vi "NI VeriStand - Save Configuration File.vi"(8 "Error in":errorcluster, 11 "Runtime Configuration Ref in":refnum<k39>) -> (0 "Error out":errorcluster, 2 "Success":bool, 3 "Runtime Configuration Ref out":refnum<k39>)   [LabVIEW 2027, in "Runtime Configuration File API.lvlib"]
uses:
  Runtime Configuration File API.lvlib
  C:/NetCoreDLL/NationalInstruments.VeriStand.SystemDefinitionAPI.dll
  NetCoreDLL/NationalInstruments.VeriStand.SystemDefinitionAPI.dll
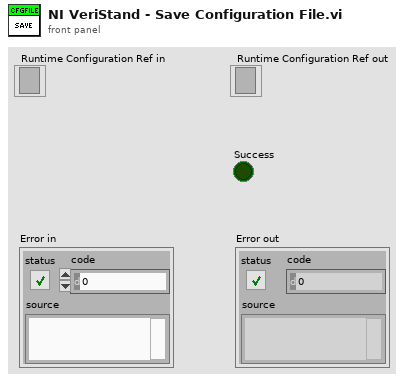
[diagram p1: front panel]
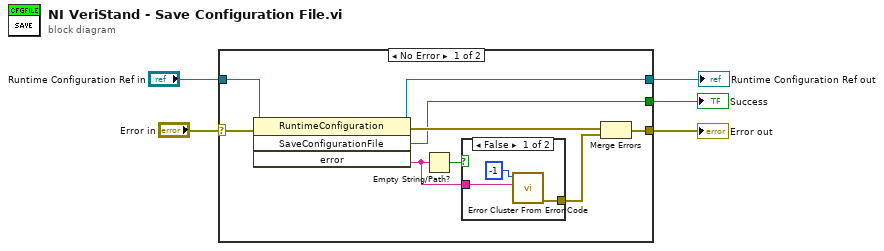
[diagram p0: block diagram]
diagram:
  n1 = case shown="No Error" "Error in" {
    selector: "Error in" -> [w14 _]
    tunnel: "Runtime Configuration Ref in" -> [w10 w18]
    tunnel: [w9 w18] -> w2
    tunnel: [w8 _] -> w1
    tunnel: [w12 _] -> w5
    frame No Error {
      n2 = invoke class="RuntimeConfiguration" method="SaveConfigurationFile"(reference=w10, error in=w14) -> (reference out=w9:refnum<k39>, error out=w11:errorcluster, "SaveConfigurationFile"=w8:bool, "error"=w6:string)  [unwired: 2 in]
      n3 = Empty String/Path?(string/path=w6) -> (empty?=w7:bool)
      n4 = case shown="False" w7 {
        tunnel: [w17 _] -> w13
        tunnel: w6 -> [w16 _]
        frame False {
          n5 = call <vilib>:"Error Cluster From Error Code.vi"("error message (\"\")"=w16, "error code (0)"=-1) -> ("error out"=w17:errorcluster)  [unwired: 7 in]
        }
        frame True {
        }
      }
      n6 = Merge Errors(w11, w13) -> (w12:errorcluster)
    }
    frame Error {
    }
  }
  "Runtime Configuration Ref out" <- w2
  "Success" <- w1
  "Error out" <- w5
